vi "Lex InvertedSection-Text.vi"(8 "Error In":errorcluster) -> (0 "Error Out":errorcluster)   [LabVIEW 2018, in "Tests.lvlib" / "Lexer.lvlib"]
uses:
  Lexer.lvlib
  <vilib>/addons/_JKI Toolkits/Caraya/classes/Test/Test.lvclass
  <vilib>/addons/_JKI Toolkits/Caraya/classes/Assert/Assert.lvclass
  src/Toolkit/Low-Level/Tokens/Text/Text.lvclass
  Tests.lvlib
  src/Toolkit/Low-Level/Tokens/Token/Token.lvclass
  src/Toolkit/Low-Level/Tokens/InvertedSection/InvertedSection.lvclass
  src/Toolkit/Low-Level/Support/Lex String.vi
  D:/Users/cfield/Code/Field R&D Services/Labstache/src/Toolkit/Low-Level/Tokens/Contentable/Contentable.lvclass
  D:/Users/cfield/Code/Field R&D Services/Labstache/src/Toolkit/Low-Level/Tokens/Token/Token.lvclass
  D:/Users/cfield/Code/Field R&D Services/Labstache/src/Toolkit/Low-Level/Tokens/Keyable/Keyable.lvclass
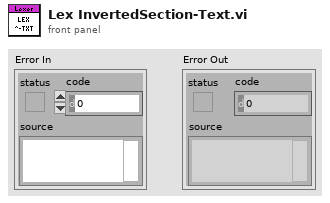
[diagram p1: front panel]
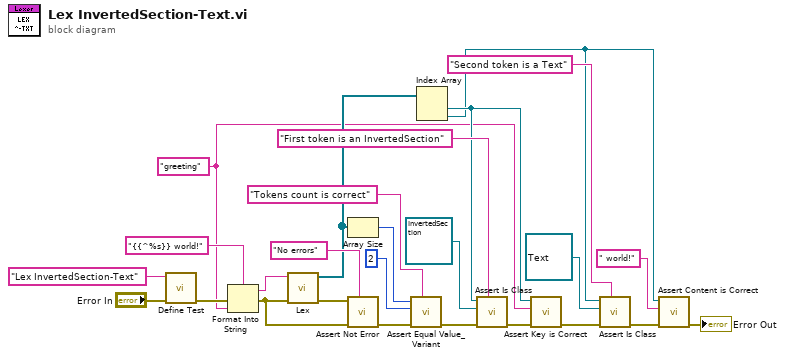
[diagram p0: block diagram]
diagram:
  w6 = "greeting" ("String")
  n1 = call <vilib>:"Define Test.vi"("error in (no error)"="Error In", "Label (VI Title)"="Lex InvertedSection-Text") -> ("error out"=w23:errorcluster)  [unwired: 9 in]
  n2 = Format Into String(format string="{{^%s}} world!", error in=w23, w6) -> (resulting string=w1:string, error out=w2:errorcluster)  [unwired: 1 in]
  n3 = call-poly "Lex.vi"("Error In"=w2, "Input"=w1) -> ("Error Out"=w24:errorcluster, "Tokens"=w17:refnum<class "Token.lvclass">[])  [unwired: 8 in]
  n4 = Array Size(array=w17) -> (size(s)=w19:i32)
  n5 = call <vilib>:"Assert Not Error.vi"("Label"="No errors", "error in (no error)"=w2, "Not Error?"=w24) -> ("error out"=w21:errorcluster)  [unwired: 8 in]
  n6 = call <vilib>:"Assert Equal Value_Variant.vi"("Label"="Tokens count is correct", "error in (no error)"=w21, "Y"=2 ("size(s)"), "X"=w19) -> ("error out"=w10:errorcluster)  [unwired: 7 in]
  n7 = Index Array(array=w17) -> (element #1=w7:refnum<class "Token.lvclass">, element #2=w4:refnum<class "Token.lvclass">)  [unwired: 2 in]
  n8 = call "Assert Is Class.vi"("Label"="First token is an InvertedSection", "Error In"=w10, "Expected"=refnum<class "InvertedSection.lvclass"> refnum ("Mustache.lvlib:Tokens.lvlib:InvertedSection.lvclass"), "Actual"=w7) -> ("Error Out"=w15:errorcluster)  [unwired: 7 in]
  n9 = call "Assert Key is Correct.vi"("Error In"=w15, "Expected"=w6, "Token"=w7) -> ("Error Out"=w9:errorcluster)  [unwired: 8 in]
  n10 = call "Assert Is Class.vi"("Label"="Second token is a Text", "Error In"=w9, "Expected"=refnum<class "Text.lvclass"> refnum ("Mustache.lvlib:Tokens.lvlib:Text.lvclass"), "Actual"=w4) -> ("Error Out"=w13:errorcluster)  [unwired: 7 in]
  n11 = call "Assert Content is Correct.vi"("Error In"=w13, "Expected"=" world!", "Token"=w4) -> ("Error Out"=→"Error Out":errorcluster)  [unwired: 8 in]
